vi "Init.vi"(8 "error in (no error)":errorcluster, 11 "Scene Name":string) -> (0 "error out":errorcluster, 3 "SetCurrentProgramScene out":refnum<class "SetCurrentProgramScene.lvclass">)   [LabVIEW 2020, in "obs-websocket.lvlib" / "SetCurrentProgramScene.lvclass"]
uses:
  SetCurrentProgramScene.lvclass
  SetCurrentProgramScene.lvclass/SetCurrentProgramScene.ctl
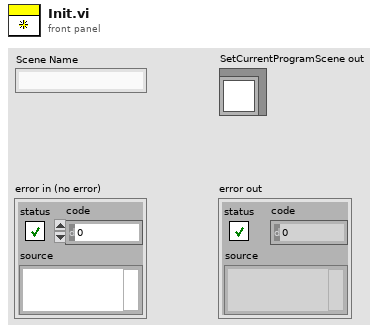
[diagram p1: front panel]
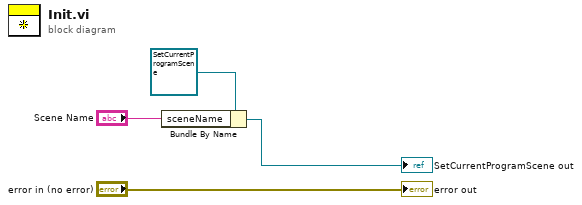
[diagram p0: block diagram]
diagram:
  n1 = Bundle By Name(cluster=refnum<class "SetCurrentProgramScene.lvclass"> refnum ("SetCurrentProgramScene in"), "sceneName"="Scene Name") -> (→"SetCurrentProgramScene out":refnum<class "SetCurrentProgramScene.lvclass">)
  "error out" <- "error in (no error)"
